vi "motor-delay.vi"() -> ()   [LabVIEW 2014]
panel:
  out "Waveform Chart":u32(graph)=18
  out "delay (ms)":u32=18
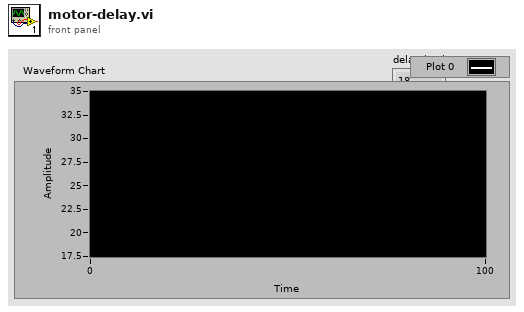
[diagram p1: front panel]
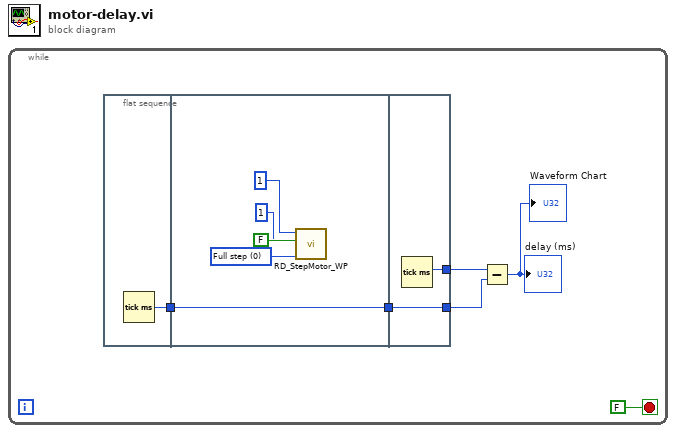
[diagram p0: block diagram]
diagram:
  n1 = while {
    stop <- FALSE stop-if-true
    n2 = flat-sequence {
      tunnel: [w7] -> w6
      tunnel: w6 -> [w8]
      tunnel: [w8] -> w5
      tunnel: [w14] -> w4
      tunnel: [w13] -> w3
      tunnel: w5 -> [w13]
      frame #0 {
        n3 = Tick Count (ms)() -> (millisecond timer value=w7:u32)
      }
      frame #1 {
        w12 = u16 0 items=["Full step", "Half step", "1/4 step", "1/8 step", "1/16 step", "1/32 step"] ("Step resolution")
        n4 = call "RD_StepMotor_WP.vi"("Step resolution"=w12, "Direction"=FALSE, "Time between steps (ms)"=1, "Steps"=i64 1) -> ()  [unwired: 8 in]
      }
      frame #2 {
        n5 = Tick Count (ms)() -> (millisecond timer value=w14:u32)
      }
    }
    n6 = Subtract(x=w4, y=w3) -> (x-y=→"delay (ms)" →"Waveform Chart":u32)
  }
